vi "ST Begin.vi"(0 "VISA resource name in":refnum<visa-resource-name>, 1 "error in":errorcluster) -> (2 "VISA resource name out":refnum<visa-resource-name>, 3 "Begin Complete":bool, 4 "error out":errorcluster)   [LabVIEW 2009]
doc: "This VI calls sends a series of commands to the ST Robot to bring it to a READY TO RUN condition.\nBEGIN COMPLETE is True if routine ran successfully"
panel:
  out "ERROR OCCURED\nFINISHED":bool
  out "HOME\nCOMPLETE":bool
  out "CALIBRATE\nCOMPLETE":bool
  out "JOINT\nCOMPLETE":bool
  out "START\nCOMPLETE":bool
  out "DECIMAL\nCOMPLETE":bool
  out "ROBOFORTH\nCOMPLETE":bool
  out "COM PORT\nWORKING":bool
  out "PURGE \nCOMPLETE":bool
  out "WHERE COMPLETE\nFINISHED":bool
  out "HOME POSITION":string
  out "CALIBRATION\nVALUES":string
  out "String Received":string
  # "THIS IS THE INITIALIZATION ROUTINE FOR THE ST R17 ROBOT"
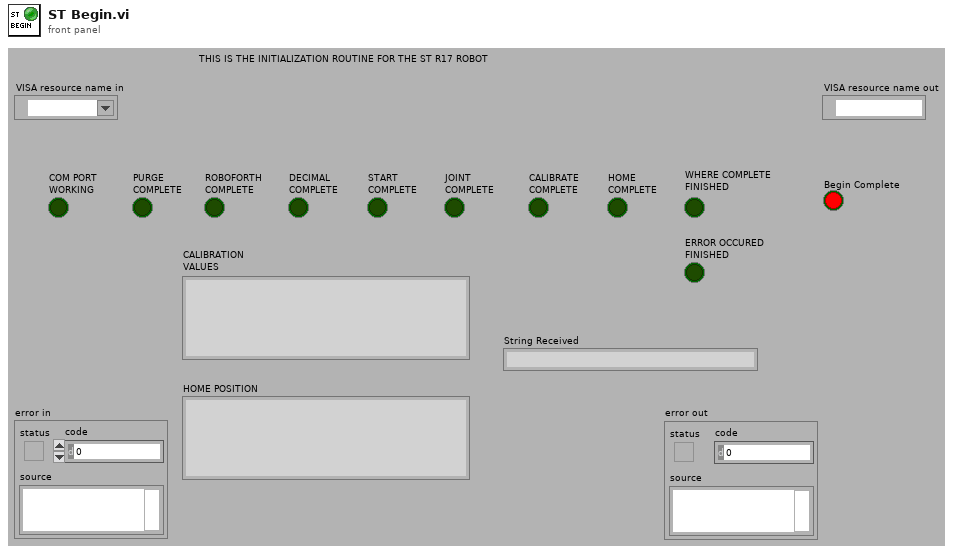
[diagram p1: front panel]
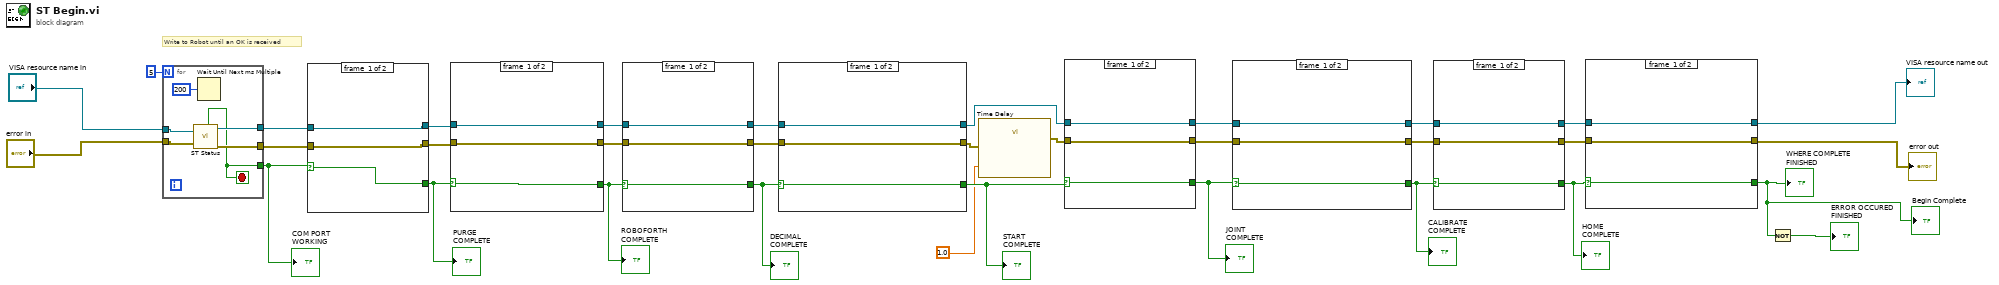
[diagram p0: block diagram]
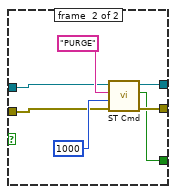
[diagram p2: hidden frame]
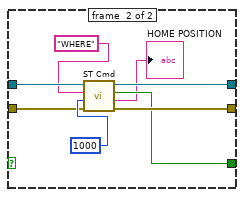
[diagram p3: hidden frame]
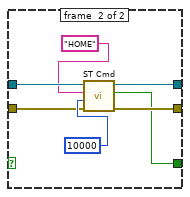
[diagram p4: hidden frame]
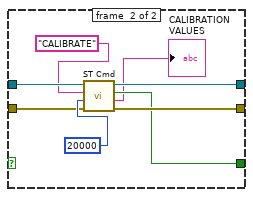
[diagram p5: hidden frame]
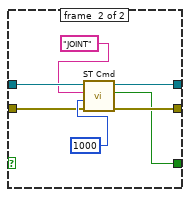
[diagram p6: hidden frame]
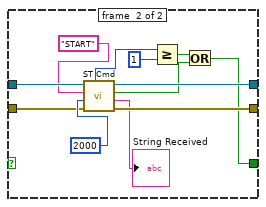
[diagram p7: hidden frame]
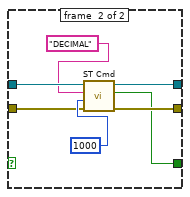
[diagram p8: hidden frame]
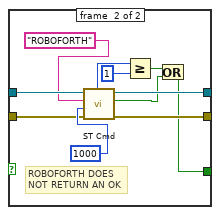
[diagram p9: hidden frame]
diagram:
  # "Write to Robot until an OK is received"
  n1 = for {
    N: 5 -> [_]
    tunnel: "VISA resource name in" -> [w38]
    tunnel: "error in" -> [w39]
    tunnel: [w37] -> w18
    tunnel: [w36] -> w19
    tunnel: [w34] -> w16
    stop <- w34 stop-if-true
    n2 = call "ST Status.vi"("error in (no error)"=w39, "VISA resource name"=w38) -> ("error out"=w37:errorcluster, "VISA resource name out"=w36:refnum<visa-resource-name>, "Ready and OK"=w34:bool)  [unwired: 2 out]
    n3 = Wait Until Next ms Multiple(millisecond multiple=u32 200) -> ()  [unwired: 1 out]
  }
  "COM PORT\nWORKING" <- w16
  n4 = case shown="True" w16 {
    selector: w16 -> [w40 _]
    tunnel: [w42 w49] -> w33
    tunnel: [w41 w48] -> w32
    tunnel: [w40 w47] -> w31
    tunnel: w19 -> [w42 w44]
    tunnel: w18 -> [w41 w43]
    frame #0 {
    }
    frame #1 {
      n5 = call "ST Cmd.vi"("error in (no error)"=w43, "Time Out"=1000, "Command String"="PURGE", "VISA resource name"=w44) -> ("error out"=w48:errorcluster, "Ready and OK"=w47:bool, "VISA resource name out"=w49:refnum<visa-resource-name>)  [unwired: 2 out]
    }
  }
  "PURGE \nCOMPLETE" <- w31
  n6 = case shown="True" w31 {
    selector: w31 -> [w50 _]
    tunnel: w33 -> [w52 w62]
    tunnel: w32 -> [w51 w61]
    tunnel: [w52 w59] -> w30
    tunnel: [w51 w58] -> w29
    tunnel: [w50 w53] -> w28
    frame #0 {
    }
    frame #1 {
      # "ROBOFORTH DOES\nNOT RETURN AN OK"
      n7 = call "ST Cmd.vi"("error in (no error)"=w61, "Time Out"=1000, "Command String"="ROBOFORTH", "VISA resource name"=w62) -> ("error out"=w58:errorcluster, "Ready and OK"=w54:bool, "VISA resource name out"=w59:refnum<visa-resource-name>, "Result Code"=w57:i32)  [unwired: 1 out]
      n8 = Greater Or Equal?(x=w57, y=1) -> (x >= y?=w55:bool)
      n9 = Or(x=w55, y=w54) -> (x .or. y?=w53:bool)
    }
  }
  "ROBOFORTH\nCOMPLETE" <- w28
  n10 = case shown="True" w28 {
    selector: w28 -> [w64 _]
    tunnel: w30 -> [w66 w72]
    tunnel: w29 -> [w65 w71]
    tunnel: [w66 w69] -> w27
    tunnel: [w65 w68] -> w26
    tunnel: [w64 w67] -> w15
    frame #0 {
    }
    frame #1 {
      n11 = call "ST Cmd.vi"("error in (no error)"=w71, "Time Out"=1000, "Command String"="DECIMAL", "VISA resource name"=w72) -> ("error out"=w68:errorcluster, "Ready and OK"=w67:bool, "VISA resource name out"=w69:refnum<visa-resource-name>)  [unwired: 2 out]
    }
  }
  "DECIMAL\nCOMPLETE" <- w15
  n12 = case shown="True" w15 {
    selector: w15 -> [w74 _]
    tunnel: w27 -> [w76 w87]
    tunnel: w26 -> [w75 w86]
    tunnel: [w76 w84] -> w8
    tunnel: [w75 w83] -> w10
    tunnel: [w74 w77] -> w14
    frame #0 {
    }
    frame #1 {
      n13 = call "ST Cmd.vi"("error in (no error)"=w86, "Time Out"=2000, "Command String"="START", "VISA resource name"=w87) -> ("error out"=w83:errorcluster, "String Received"=→"String Received":string, "Ready and OK"=w78:bool, "VISA resource name out"=w84:refnum<visa-resource-name>, "Result Code"=w79:i32)
      n14 = Greater Or Equal?(x=w79, y=1) -> (x >= y?=w80:bool)
      n15 = Or(x=w80, y=w78) -> (x .or. y?=w77:bool)
    }
  }
  "START\nCOMPLETE" <- w14
  n16 = call "Time Delay"("error in (no error)"=w10, "Delay Time (s)"=1.0) -> ("error out"=w9:errorcluster)  [unwired: 9 in]
  n17 = case shown="True" w14 {
    selector: w14 -> [w89 _]
    tunnel: w8 -> [w91 w97]
    tunnel: w9 -> [w90 w96]
    tunnel: [w91 w94] -> w25
    tunnel: [w90 w93] -> w24
    tunnel: [w89 w92] -> w13
    frame #0 {
    }
    frame #1 {
      n18 = call "ST Cmd.vi"("error in (no error)"=w96, "Time Out"=1000, "Command String"="JOINT", "VISA resource name"=w97) -> ("error out"=w93:errorcluster, "Ready and OK"=w92:bool, "VISA resource name out"=w94:refnum<visa-resource-name>)  [unwired: 2 out]
    }
  }
  "JOINT\nCOMPLETE" <- w13
  n19 = case shown="True" w13 {
    selector: w13 -> [w99 _]
    tunnel: w25 -> [w101 w108]
    tunnel: w24 -> [w100 w107]
    tunnel: [w101 w105] -> w23
    tunnel: [w100 w104] -> w22
    tunnel: [w99 w103] -> w12
    frame #0 {
    }
    frame #1 {
      n20 = call "ST Cmd.vi"("error in (no error)"=w107, "Time Out"=20000, "Command String"="CALIBRATE", "VISA resource name"=w108) -> ("error out"=w104:errorcluster, "String Received"=→"CALIBRATION\nVALUES":string, "Ready and OK"=w103:bool, "VISA resource name out"=w105:refnum<visa-resource-name>)  [unwired: 1 out]
    }
  }
  "CALIBRATE\nCOMPLETE" <- w12
  n21 = case shown="True" w12 {
    selector: w12 -> [w110 _]
    tunnel: w23 -> [w112 w118]
    tunnel: w22 -> [w111 w117]
    tunnel: [w112 w115] -> w21
    tunnel: [w111 w114] -> w20
    tunnel: [w110 w113] -> w11
    frame #0 {
    }
    frame #1 {
      n22 = call "ST Cmd.vi"("error in (no error)"=w117, "Time Out"=10000, "Command String"="HOME", "VISA resource name"=w118) -> ("error out"=w114:errorcluster, "Ready and OK"=w113:bool, "VISA resource name out"=w115:refnum<visa-resource-name>)  [unwired: 2 out]
    }
  }
  "HOME\nCOMPLETE" <- w11
  n23 = case shown="True" w11 {
    selector: w11 -> [w120 _]
    tunnel: w21 -> [w122 w129]
    tunnel: w20 -> [w121 w128]
    tunnel: [w122 w126] -> w4
    tunnel: [w121 w125] -> w3
    tunnel: [w120 w124] -> w1
    frame #0 {
    }
    frame #1 {
      n24 = call "ST Cmd.vi"("error in (no error)"=w128, "Time Out"=1000, "Command String"="WHERE", "VISA resource name"=w129) -> ("error out"=w125:errorcluster, "String Received"=→"HOME POSITION":string, "Ready and OK"=w124:bool, "VISA resource name out"=w126:refnum<visa-resource-name>)  [unwired: 1 out]
    }
  }
  "VISA resource name out" <- w4
  "error out" <- w3
  "Begin Complete" <- w1
  "WHERE COMPLETE\nFINISHED" <- w1
  n25 = Not(x=w1) -> (.not. x?=→"ERROR OCCURED\nFINISHED":bool)
